vi "SENS_CORR_COLL_APPL.vi"(0 "VISA IN":refnum<visa-resource-name>, 5 "error in":errorcluster, 7 "Channel":i32=1) -> (14 "VISA Out":refnum<visa-resource-name>, 19 "error out":errorcluster)   [LabVIEW 2018, in "PNA-X.lvlib"]
doc: "SENSe<cnum>:CORRection:COLLect:APPLy \n(Write-only) Applies error terms to the measurement that is selected using Calc:Par:Select. \nNote: Before using this command you must select a measurement using CALC:PAR:SEL. You can \nselect one measurement for each channel. \nNote: This command is only necessary if you need to modify error terms. If you do not need to modify \nerror terms, SENSe<cnum>:CORRection:COLLect:SAVE calculates and then automatically applies \nerror terms after you use SENS:CORR:COLL:ACQuire to measure cal standards. \nParameters \n<cnum> Any existing channel number. If unspecified, value is set to 1 \nExample CALCulate2:PARameter:SELect S21_2 'select the measurement to \napply terms to \n1. \nSENSe2:CORRection:COLLect:METHod SPARSOLT 'set type of cal \nmethod. \n2. \nCALCulate2:DATA? SCORR1 'download the error term of interest 3. \n'Modify the error term here 4. \nCALCulate2:DATA SCORR1 'upload the error term of interest 5. \nSENSe2:CORRection:COLLect:APPLy 'applies the error terms to \nthe measurement \n6. \nQuery Syntax Not applicable \nDefault Not applicable \n1628\n\nSENSe:CORRection:COLLect:ISOLation:AVERage:INCRement <num> \n(Read-Write) Specifies amount to increment (increase) the channel averaging factor during isolation \nmeasurement of the ECal module during an unguided ECal calibration. \nNote: if the channel currently has averaging turned OFF and <num> is greater than 1, averaging will \nbe turned ON only during the isolation measurements and with the averaging factor equal to <num>. \nParameters \n<num> Incremental Averaging factor. The maximum averaging factor is 65536 (2^16). \nExamples SENS:CORR:COLL:ISOL:AVER:INCR 16 \nsense:correction:collect:isolation:average:increment 0 \nQuery Syntax SENSe:CORRection:COLLect:ISOLation:AVERage:INCRement? \nReturn Type Numeric \nDefault 8 - If this command is NOT sent, but ECal isolation is measured, then \naveraging will be turned ON with factor set to 8 during the isolation \nmeasurement."
uses:
  PNA-X.lvlib
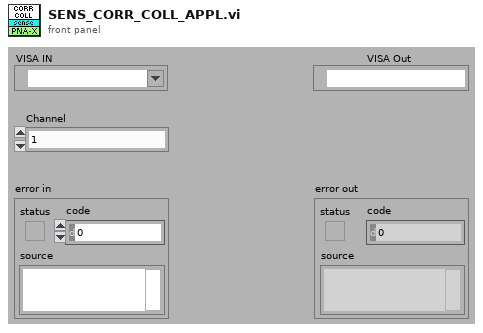
[diagram p1: front panel]
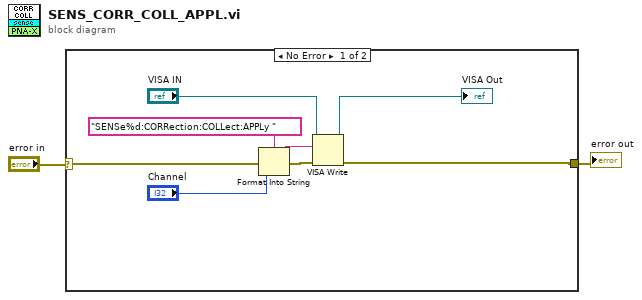
[diagram p0: block diagram]
diagram:
  n1 = case shown="No Error" "error in" {
    selector: "error in" -> [w10 w11]
    tunnel: [w5 w11] -> w1
    frame No Error {
      n2 = Format Into String(format string="SENSe%d:CORRection:COLLect:APPLy " ("Cmdline"), error in=w10, "Channel") -> (resulting string=w8:string, error out=w9:errorcluster)  [unwired: 1 in]
      n3 = VISA Write(VISA resource name="VISA IN", write buffer=w8, error in (no error)=w9) -> (VISA resource name out=→"VISA Out":refnum<visa-resource-name>, error out=w5:errorcluster)  [unwired: 1 out]
    }
    frame Error {
    }
  }
  "error out" <- w1
